vi "mp285_RelMove.vi"() -> ()   [LabVIEW 2016]
panel:
  in  "Z 2":dbl
  in  "Y 2":dbl
  in  "X 2":dbl
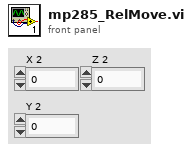
[diagram p1: front panel]
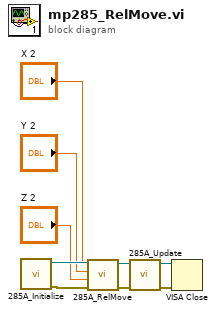
[diagram p0: block diagram]
diagram:
  n1 = call "285A_Initialize.vi"() -> ("错误输出"=w6:errorcluster, "VISA资源名称输出"=w9:refnum<visa-resource-name>)  [unwired: 10 in]
  n2 = call "285A_RelMove.vi"("VISA资源名称"=w9, "error in (no error)"=w6, "Z 2"="Z 2", "Y 2"="Y 2", "X 2"="X 2") -> ("error out"=w5:errorcluster, "VISA resource name out 2"=w8:refnum<visa-resource-name>)  [unwired: 1 in, 4 out]
  n3 = call "285A_Update.vi"("错误输入（无错误）"=w5, "VISA资源名称"=w8) -> ("error out"=w4:errorcluster, "VISA资源名称 2"=w7:refnum<visa-resource-name>)  [unwired: 8 in]
  n4 = VISA Close(VISA resource name=w7, error in (no error)=w4) -> ()  [unwired: 1 out]
